vi "io_bin_data_PC_to_instrument.vi"(5 "Binary Data":string, 8 "error in":errorcluster, 10 "Command (none)":string, 11 "VISA resource name":refnum<visa-resource-name>) -> (0 "error out":errorcluster, 3 "VISA resource name out":refnum<visa-resource-name>)   [LabVIEW 2014, in "rszvl_rsidr_core.lvlib"]
uses:
  rszvl_rsidr_core.lvlib
  type_Error_Codes.ctl
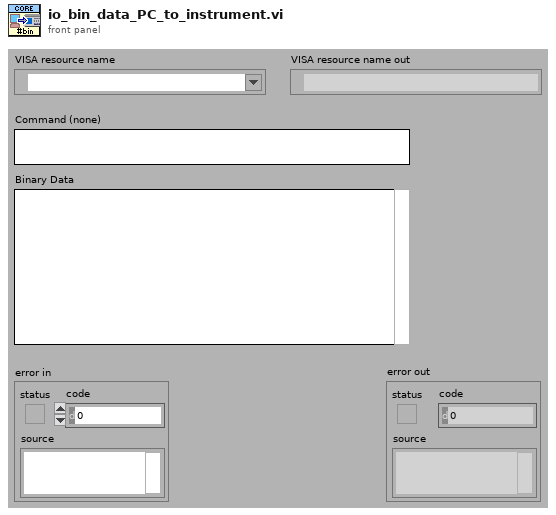
[diagram p1: front panel]
types:
  T1 = typedef "rszvl_rsidr_core.lvlib/type_Error_Codes.ctl" = enum16{"No_error", "VISA_err_ResourceNotFound", "VISA_err_Timeout", "VISA_warn_MoreDataAvailable", "RS_err_MissingCallback", "RS_err_InvalidAttribute", "RS_err_InvalidValue", "RS_err_UnknownResource", "RS_err_AlreadyInitialized", "RS_err_InstrumentStatus", "RS_err_BadRepCapName", "RS_err_TypesMismatch", "RS_err_ValueNotSupported", "RS_err_InvalidRngTable", "RS_err_IDqueryFail", "RS_err_UnexpResponse", "VISA_warn_ConfigNotLoaded", "RS_err_AttributeNotReadable", "RS_err_AttributeNotWritable", "RS_err_InstrumentType", "RS_err_InstrumentOption", "VISA_err_InvalidSize", "RS_err_ReliabilityIndicator", "VISA_warn_UnknownStatus", "VISA_warn_TermCharRead", "VISA_err_IO_error"}
  T2 = typedef "rszvl_rsidr_core.lvlib/type_Session_Data.ctl" = cluster{"Instr type":string, "Instr type for err. msg.":string, "Installed Options":string[], "OPC Timeout":i32, "Query Instrument Status":bool, "Check Range":bool, "Check Options":bool, "Add LF to Write":bool, "Simulate":bool, "Logging":bool, "Logging params":variant, "Interface Type":enum16{"Unknown", "GPIB", "VXI", "GPIB_VXI", "ASRL", "PXI", "TCPIP", "USB", "SOCKET"}, "Fast Sweep":i32, "AdditionalFlags":i32, "WaitBeforeWrite":i32, "WaitBeforeRead":i32, "BinDataChunkSize":i64}
  T3 = enum16{"Unknown", "GPIB", "VXI", "GPIB_VXI", "ASRL", "PXI", "TCPIP", "USB", "SOCKET"}
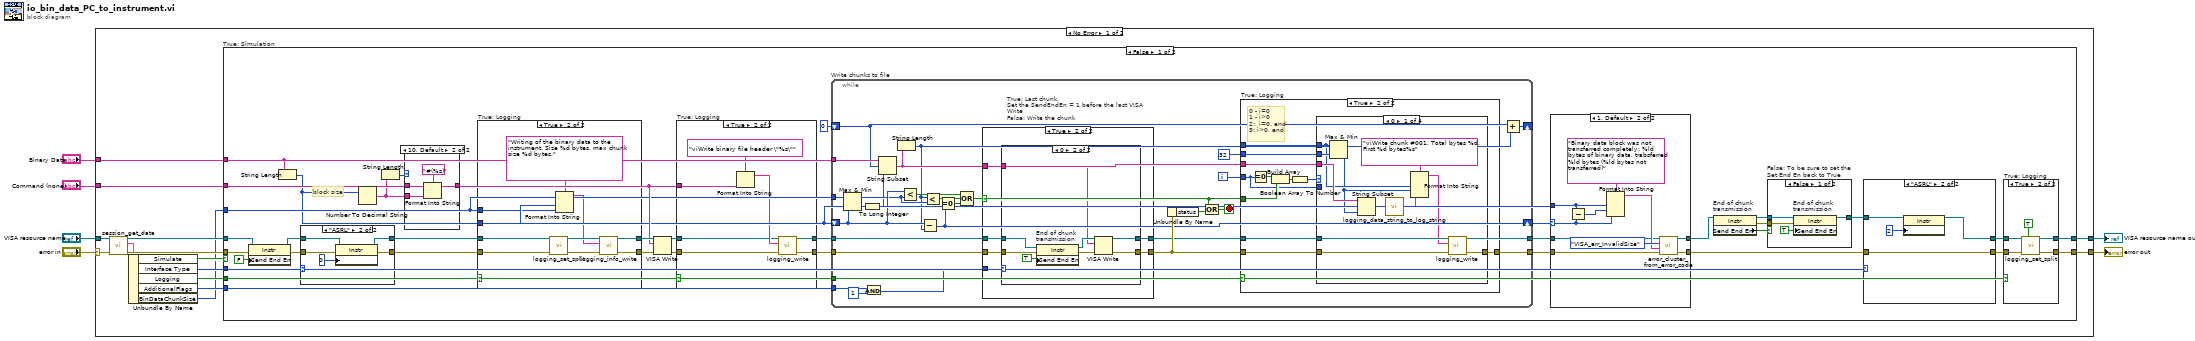
[diagram p0: block diagram]
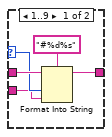
[diagram p7: hidden frame]
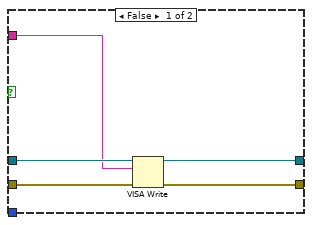
[diagram p8: hidden frame]
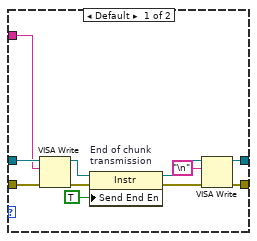
[diagram p9: hidden frame]
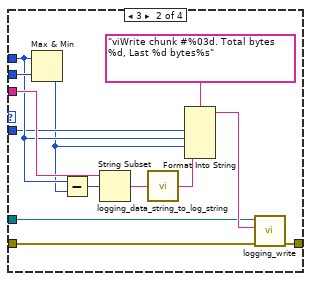
[diagram p11: hidden frame]
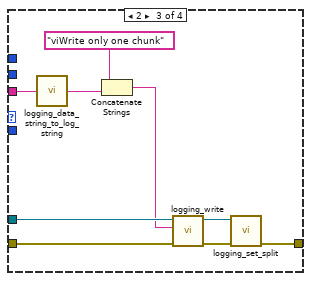
[diagram p12: hidden frame]
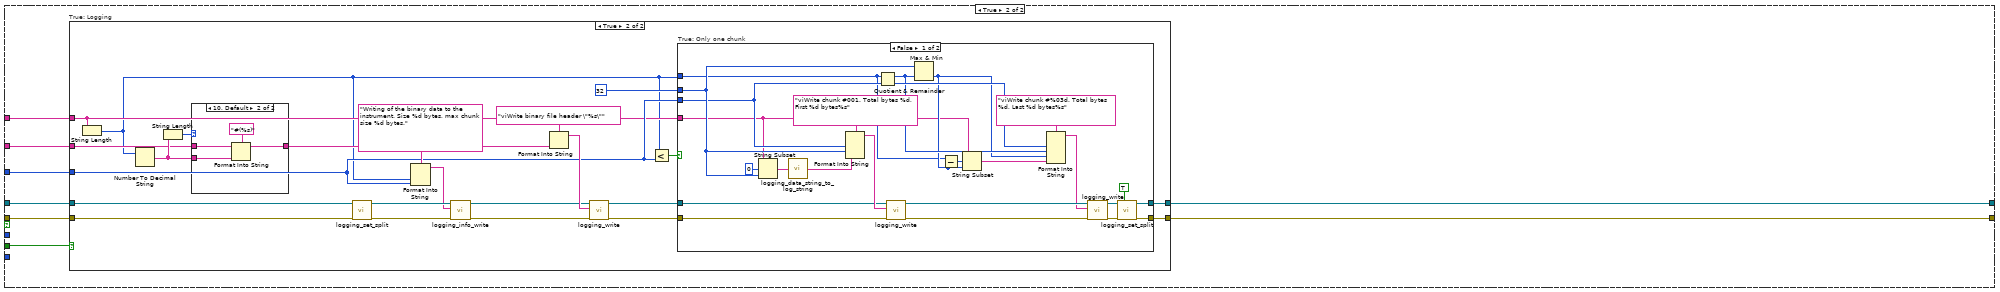
[diagram p16: hidden frame]
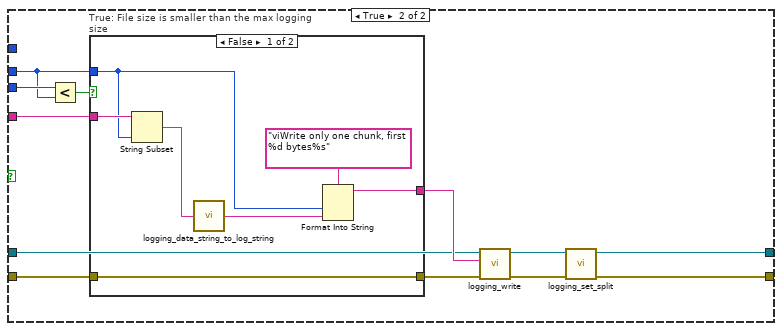
[diagram p18: hidden frame]
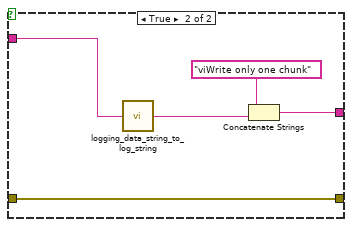
[diagram p19: hidden frame]
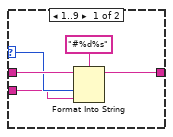
[diagram p20: hidden frame]
diagram:
  n1 = case shown="No Error" "error in" {
    selector: "error in" -> [w18 w319]
    tunnel: "Binary Data" -> [w20 _]
    tunnel: "Command (none)" -> [w19 _]
    tunnel: "VISA resource name" -> [w17 w320]
    tunnel: [w12 w319] -> w3
    tunnel: [w11 w320] -> w2
    frame No Error {
      n2 = call "session_get_data.vi"("error in"=w18, "VISA resource name"=w17) -> ("error out"=w16:errorcluster, "Session User Data out"=w14:T2, "VISA resource name out"=w15:refnum<visa-resource-name>)  [unwired: 7 in]
      n3 = Unbundle By Name(w14) -> ("Simulate"=w10:bool, "Interface Type"=w9:T3, "Logging"=w13:bool, "AdditionalFlags"=w8:i32, "BinDataChunkSize"=w7:i64)
      n4 = case "True: Simulation" shown="False" w10 {
        tunnel: w16 -> [w30 w232]
        tunnel: w15 -> [w57 w231]
        tunnel: w20 -> [w29 w230]
        tunnel: w19 -> [w53 w229]
        tunnel: [w37 w233] -> w11
        tunnel: [w27 w234] -> w12
        tunnel: w13 -> [w40 w235]
        tunnel: w7 -> [w41 w228]
        tunnel: w9 -> [w32 _]
        tunnel: w8 -> [w31 _]
        frame False {
          # "block size"
          n5 = property on="Property Node" class="Instr"(reference=w57, error in=w30, "Send End En"=FALSE ("Message Based Settings:Send End Enable")) -> (reference out=w54:refnum<visa-resource-name>, error out=w55:errorcluster)
          n6 = String Length(string=w29) -> (length=w21:i32)
          n7 = case "4: ASRL" shown="\"ASRL\"" w32 {
            tunnel: w55 -> [w221 w226]
            tunnel: w54 -> [w222 w225]
            tunnel: [w222 w224] -> w50
            tunnel: [w221 w223] -> w49
            frame Default {
            }
            frame "ASRL" {
              n8 = property on="Property Node" class="Instr"(reference=w225, error in=w226, "Serial Settings:End Mode for Reads"=u16 0 ("ASRL End In")) -> (reference out=w224:refnum<visa-resource-name>, error out=w223:errorcluster)
            }
          }
          n9 = Number To Decimal String(number=w21) -> (decimal integer string=w52:string)  [unwired: 1 in]
          n10 = String Length(string=w52) -> (length=w51:i32)
          n11 = case shown="10, Default" w51 {
            selector: w51 -> [w105 _]
            tunnel: w53 -> [w106 w110]
            tunnel: w52 -> [w104 w108]
            tunnel: [w103 w109] -> w43
            frame 1..9 {
              n12 = Format Into String(format string="#%d%s", initial string=w106, w105, w104) -> (resulting string=w103:string)  [unwired: 1 in, 1 out]
            }
            frame 10, Default {
              n13 = Format Into String(format string="#(%s)", initial string=w110, w108) -> (resulting string=w109:string)  [unwired: 1 in, 1 out]
            }
          }
          n14 = case "True: Logging" shown="True" w40 {
            tunnel: w49 -> [w92 w102]
            tunnel: w50 -> [w91 w101]
            tunnel: w41 -> [_ w98]
            tunnel: [w92 w95] -> w47
            tunnel: [w91 w94] -> w48
            tunnel: w21 -> [_ w99]
            frame False {
            }
            frame True {
              n15 = call "logging_set_split.vi"("error in"=w102, "VISA resource name"=w101) -> ("error out"=w97:errorcluster, "VISA resource name out"=w96:refnum<visa-resource-name>)  [unwired: 8 in]
              n16 = Format Into String(format string="Writing of the binary data to the instrument. Size %d bytes, max chunk size %d bytes.", w99, w98) -> (resulting string=w93:string)  [unwired: 2 in, 1 out]
              n17 = call "logging_info_write.vi"("error in"=w97, "String to write"=w93, "VISA resource name"=w96) -> ("error out"=w95:errorcluster, "VISA resource name out"=w94:refnum<visa-resource-name>)  [unwired: 7 in]
            }
          }
          n18 = VISA Write(VISA resource name=w48, write buffer=w43, error in (no error)=w47) -> (VISA resource name out=w45:refnum<visa-resource-name>, error out=w46:errorcluster)  [unwired: 1 out]
          n19 = case "True: Logging" shown="True" w40 {
            tunnel: w46 -> [w83 w88]
            tunnel: w45 -> [w82 w87]
            tunnel: [w83 w86] -> w44
            tunnel: [w82 w85] -> w42
            tunnel: w43 -> [_ w84]
            frame False {
            }
            frame True {
              n20 = Format Into String(format string="viWrite binary file header \"%s\"", w84) -> (resulting string=w89:string)  [unwired: 2 in, 1 out]
              n21 = call "logging_write.vi"("error in"=w88, "String to write"=w89, "VISA resource name"=w87) -> ("error out"=w86:errorcluster, "VISA resource name out"=w85:refnum<visa-resource-name>)  [unwired: 7 in]
            }
          }
          n22 = while "Write chunks to file" {
            tunnel: w44 -> [w118]
            tunnel: w42 -> [w127]
            tunnel: w41 -> [w134]
            shift-right: [w113] -> w25
            shift-left: w21 -> [w136]
            tunnel: [w133] -> w24
            tunnel: w40 -> [w131]
            tunnel: [w125] -> w26
            tunnel: w31 -> [w122]
            tunnel: w29 -> [w120]
            shift-right: [w116] -> _
            shift-left: 0 -> [w115]
            i -> [w128]
            stop <- w137 stop-if-true
            n23 = Max & Min(x=w134, y=w136) -> (min(x,y)=w135:i64)  [unwired: 1 out]
            n24 = To Long Integer(number=w135) -> (32bit integer=w119:i32)
            n25 = And(x=w122, y=1 ("x")) -> (x .and. y?=w121:i32)
            n26 = String Subset(string=w120, offset (0)=w115, length (rest)=w119) -> (substring=w117:string)
            n27 = String Length(string=w117) -> (length=w114:i32)
            n28 = Less?(x=w136, y=w134) -> (x < y?=w130:bool)
            n29 = Subtract(x=w136, y=w114) -> (x-y=w113:i32)
            n30 = Less?(x=w114, y=w134) -> (x < y?=w129:bool)
            n31 = Equal To 0?(x=w113) -> (x = 0?=w112:bool)
            n32 = Compound Arithmetic op=OR(w130, w129, w112) -> (w124:bool)
            n33 = case "True: Last chunk,\nSet the SendEndEn = 1 before the last VISA Write\nFalse: Write the chunk" shown="True" w124 {
              tunnel: w127 -> [w142 w149]
              tunnel: w118 -> [w143 w148]
              tunnel: [w141 w147] -> w126
              tunnel: w117 -> [w139 w146]
              tunnel: [w140 w145] -> w125
              tunnel: w121 -> [_ w144]
              frame False {
                n34 = VISA Write(VISA resource name=w142, write buffer=w139, error in (no error)=w143) -> (VISA resource name out=w140:refnum<visa-resource-name>, error out=w141:errorcluster)  [unwired: 1 out]
              }
              frame True {
                n35 = case shown="0" w144 {
                  tunnel: w149 -> [w154 w168]
                  tunnel: w148 -> [w155 w167]
                  tunnel: [w158 w164] -> w147
                  tunnel: w146 -> [w151 w163]
                  tunnel: [w157 w162] -> w145
                  frame Default {
                    n36 = VISA Write(VISA resource name=w154, write buffer=w151, error in (no error)=w155) -> (VISA resource name out=w152:refnum<visa-resource-name>, error out=w153:errorcluster)  [unwired: 1 out]
                    n37 = property on="End of chunk\ntransmission" class="Instr"(reference=w152, error in=w153, "Send End En"=TRUE ("Message Based Settings:Send End Enable")) -> (reference out=w159:refnum<visa-resource-name>, error out=w160:errorcluster)
                    n38 = VISA Write(VISA resource name=w159, write buffer="\n" ("Line Feed Constant"), error in (no error)=w160) -> (VISA resource name out=w157:refnum<visa-resource-name>, error out=w158:errorcluster)  [unwired: 1 out]
                  }
                  frame 0 {
                    n39 = property on="End of chunk\ntransmission" class="Instr"(reference=w168, error in=w167, "Send End En"=TRUE ("Message Based Settings:Send End Enable")) -> (reference out=w165:refnum<visa-resource-name>, error out=w166:errorcluster)
                    n40 = VISA Write(VISA resource name=w165, write buffer=w163, error in (no error)=w166) -> (VISA resource name out=w162:refnum<visa-resource-name>, error out=w164:errorcluster)  [unwired: 1 out]
                  }
                }
              }
            }
            n41 = Unbundle By Name(w126) -> ("status"=w138:bool)
            n42 = Compound Arithmetic op=OR(w124, w138) -> (w137:bool)
            n43 = case "True: Logging" shown="True" w131 {
              tunnel: w126 -> [w169 w180]
              tunnel: w125 -> [_ w179]
              tunnel: [w169 w178] -> w133
              tunnel: w117 -> [_ w177]
              tunnel: w114 -> [_ w176]
              tunnel: 32 ("length (rest)") -> [_ w175]
              tunnel: w124 -> [_ w174]
              tunnel: w128 -> [_ w170]
              frame False {
              }
              frame True {
                # "0 - i=0\n1 - i>0\n2:  i=0, end\n3: i>0, end"
                n44 = Equal To 0?(x=w170) -> (x = 0?=w173:bool)
                n45 = Build Array(w173, w174) -> (w172:bool[])
                n46 = Boolean Array To Number(Boolean array=w172) -> (number=w171:u32)
                n47 = case shown="0" w171 {
                  tunnel: w180 -> [w189 w202 w213 w214]
                  tunnel: w179 -> [w188 w201 w212 _]
                  tunnel: [w187 w192 w205 w214] -> w178
                  tunnel: w177 -> [w186 w200 w211 _]
                  tunnel: w176 -> [w183 w197 _ _]
                  tunnel: w175 -> [w184 w198 _ _]
                  tunnel: w170 -> [_ w195 _ _]
                  frame 0 {
                    n48 = Max & Min(x=w183, y=w184) -> (min(x,y)=w182:i32)  [unwired: 1 out]
                    n49 = String Subset(string=w186, length (rest)=w182) -> (substring=w185:string)  [unwired: 1 in]
                    n50 = call "logging_data_string_to_log_string.vi"("Raw string to log"=w185) -> ("Result log string"=w181:string)  [unwired: 4 in]
                    n51 = Format Into String(format string="viWrite chunk #001. Total bytes %d, First %d bytes%s", w183, w182, w181) -> (resulting string=w190:string)  [unwired: 2 in, 1 out]
                    n52 = call "logging_write.vi"("error in"=w189, "String to write"=w190, "VISA resource name"=w188) -> ("error out"=w187:errorcluster)  [unwired: 7 in, 1 out]
                  }
                  frame 3 {
                    n53 = Max & Min(x=w197, y=w198) -> (min(x,y)=w194:i32)  [unwired: 1 out]
                    n54 = Subtract(x=w197, y=w194) -> (x-y=w196:i32)
                    n55 = String Subset(string=w200, offset (0)=w196) -> (substring=w199:string)  [unwired: 1 in]
                    n56 = call "logging_data_string_to_log_string.vi"("Raw string to log"=w199) -> ("Result log string"=w193:string)  [unwired: 4 in]
                    n57 = Format Into String(format string="viWrite chunk #%03d. Total bytes %d, Last %d bytes%s", w195, w197, w194, w193) -> (resulting string=w203:string)  [unwired: 2 in, 1 out]
                    n58 = call "logging_write.vi"("error in"=w202, "String to write"=w203, "VISA resource name"=w201) -> ("error out"=w192:errorcluster)  [unwired: 7 in, 1 out]
                  }
                  frame 2 {
                    n59 = call "logging_data_string_to_log_string.vi"("Raw string to log"=w211) -> ("Result log string"=w208:string)  [unwired: 4 in]
                    n60 = Concatenate Strings("viWrite only one chunk" ("format string"), w208) -> (w209:string)
                    n61 = call "logging_write.vi"("error in"=w213, "String to write"=w209, "VISA resource name"=w212) -> ("error out"=w207:errorcluster, "VISA resource name out"=w206:refnum<visa-resource-name>)  [unwired: 7 in]
                    n62 = call "logging_set_split.vi"("error in"=w207, "VISA resource name"=w206) -> ("error out"=w205:errorcluster)  [unwired: 8 in, 1 out]
                  }
                  frame Default {
                  }
                }
              }
            }
            n63 = Add(x=w115, y=w114) -> (x+y=w116:i32)
          }
          n64 = case shown="1, Default" w25 {
            selector: w25 -> [_ w61]
            tunnel: w26 -> [w59 w65]
            tunnel: w24 -> [w58 w64]
            tunnel: [w58 w63] -> w23
            tunnel: [w59 w62] -> w22
            tunnel: w21 -> [_ w60]
            frame 0 {
            }
            frame 1, Default {
              n65 = Subtract(x=w60, y=w61) -> (x-y=w67:i32)
              n66 = Format Into String(format string="Binary data block was not transferred completely: %ld bytes of binary data, trabsferred %ld bytes (%ld bytes not transferred)" ("error message (\"\")"), w60, w67, w61) -> (resulting string=w68:string)  [unwired: 2 in, 1 out]
              n67 = call "error_cluster_from_error_code.vi"("error in"=w64, "error message (\"\")"=w68, "Error Enum in"=type_Error_Codes."VISA_err_InvalidSize", "VISA resource name"=w65) -> ("error out"=w63:errorcluster, "VISA resource name out"=w62:refnum<visa-resource-name>)  [unwired: 6 in]
            }
          }
          n68 = property on="End of chunk\ntransmission" class="Instr"(reference=w22) -> (reference out=w36:refnum<visa-resource-name>, error out=w34:errorcluster, "Send End En"=w35:bool)  [unwired: 1 in]
          n69 = case "False: To be sure to set the\nSet End En back to True" shown="False" w35 {
            tunnel: w36 -> [w73 w74]
            tunnel: w34 -> [w72 _]
            tunnel: [w71 w74] -> w33
            frame False {
              n70 = property on="End of chunk\ntransmission" class="Instr"(reference=w73, error in=w72, "Send End En"=TRUE ("Message Based Settings:Send End Enable")) -> (reference out=w71:refnum<visa-resource-name>)  [unwired: 1 out]
            }
            frame True {
            }
          }
          n71 = case "4: ASRL" shown="\"ASRL\"" w32 {
            tunnel: w33 -> [w215 w219]
            tunnel: [w215 w217] -> w38
            tunnel: w23 -> [w216 w218]
            tunnel: [w216 w218] -> w39
            frame Default {
            }
            frame "ASRL" {
              n72 = property on="Property Node" class="Instr"(reference=w219, "Serial Settings:End Mode for Reads"=u16 2 ("ASRL End In")) -> (reference out=w217:refnum<visa-resource-name>)  [unwired: 1 in, 1 out]
            }
          }
          n73 = case "True: Logging" shown="True" w40 {
            tunnel: w39 -> [w76 w81]
            tunnel: w38 -> [w75 w80]
            tunnel: [w76 w79] -> w27
            tunnel: [w75 w78] -> w37
            frame False {
            }
            frame True {
              n74 = call "logging_set_split.vi"("Evaluate section error (F)"=TRUE, "error in"=w81, "VISA resource name"=w80) -> ("error out"=w79:errorcluster, "VISA resource name out"=w78:refnum<visa-resource-name>)  [unwired: 7 in]
            }
          }
        }
        frame True {
          n75 = case "True: Logging" shown="True" w235 {
            tunnel: w232 -> [w237 w240]
            tunnel: w231 -> [w236 w255]
            tunnel: [w237 w242] -> w234
            tunnel: [w236 w241] -> w233
            tunnel: w230 -> [_ w239]
            tunnel: w229 -> [_ w258]
            tunnel: w228 -> [_ w245]
            frame False {
            }
            frame True {
              n76 = String Length(string=w239) -> (length=w238:i32)
              n77 = Number To Decimal String(number=w238) -> (decimal integer string=w260:string)  [unwired: 1 in]
              n78 = String Length(string=w260) -> (length=w259:i32)
              n79 = case shown="10, Default" w259 {
                selector: w259 -> [w312 _]
                tunnel: w258 -> [w313 w317]
                tunnel: w260 -> [w311 w315]
                tunnel: [w310 w316] -> w248
                frame 1..9 {
                  n80 = Format Into String(format string="#%d%s", initial string=w313, w312, w311) -> (resulting string=w310:string)  [unwired: 1 in, 1 out]
                }
                frame 10, Default {
                  n81 = Format Into String(format string="#(%s)", initial string=w317, w315) -> (resulting string=w316:string)  [unwired: 1 in, 1 out]
                }
              }
              n82 = call "logging_set_split.vi"("error in"=w240, "VISA resource name"=w255) -> ("error out"=w256:errorcluster, "VISA resource name out"=w257:refnum<visa-resource-name>)  [unwired: 8 in]
              n83 = Format Into String(format string="Writing of the binary data to the instrument. Size %d bytes, max chunk size %d bytes.", w238, w245) -> (resulting string=w253:string)  [unwired: 2 in, 1 out]
              n84 = call "logging_info_write.vi"("error in"=w256, "String to write"=w253, "VISA resource name"=w257) -> ("error out"=w250:errorcluster, "VISA resource name out"=w249:refnum<visa-resource-name>)  [unwired: 7 in]
              n85 = Format Into String(format string="viWrite binary file header \"%s\"", w248) -> (resulting string=w251:string)  [unwired: 2 in, 1 out]
              n86 = call "logging_write.vi"("error in"=w250, "String to write"=w251, "VISA resource name"=w249) -> ("error out"=w244:errorcluster, "VISA resource name out"=w243:refnum<visa-resource-name>)  [unwired: 7 in]
              n87 = Less?(x=w238, y=w245) -> (x < y?=w247:bool)
              n88 = case "True: Only one chunk" shown="False" w247 {
                tunnel: 32 ("length (rest)") -> [w278 w290]
                tunnel: w239 -> [w263 w297]
                tunnel: w244 -> [w267 w293]
                tunnel: w245 -> [w277 w296]
                tunnel: w243 -> [w281 w291]
                tunnel: [w271 w287] -> w242
                tunnel: [w270 w286] -> w241
                tunnel: w238 -> [w264 _]
                frame False {
                  n89 = String Subset(string=w263, offset (0)=0, length (rest)=w278) -> (substring=w284:string)
                  n90 = call "logging_data_string_to_log_string.vi"("Raw string to log"=w284) -> ("Result log string"=w285:string)  [unwired: 4 in]
                  n91 = Format Into String(format string="viWrite chunk #001. Total bytes %d, First %d bytes%s", w277, w278, w285) -> (resulting string=w283:string)  [unwired: 2 in, 1 out]
                  n92 = Quotient & Remainder(x=w264, y=w277) -> (x-y*floor(x/y)=w274:i64, floor(x/y)=w275:i64)
                  n93 = call "logging_write.vi"("error in"=w267, "String to write"=w283, "VISA resource name"=w281) -> ("error out"=w262:errorcluster, "VISA resource name out"=w280:refnum<visa-resource-name>)  [unwired: 7 in]
                  n94 = Max & Min(x=w278, y=w274) -> (min(x,y)=w265:i64)  [unwired: 1 out]
                  n95 = Subtract(x=w264, y=w265) -> (x-y=w266:i64)
                  n96 = String Subset(string=w263, offset (0)=w266, length (rest)=w265) -> (substring=w261:string)
                  n97 = Format Into String(format string="viWrite chunk #%03d. Total bytes %d, Last %d bytes%s", w275, w274, w265, w261) -> (resulting string=w276:string)  [unwired: 2 in, 1 out]
                  n98 = call "logging_write.vi"("error in"=w262, "String to write"=w276, "VISA resource name"=w280) -> ("error out"=w273:errorcluster, "VISA resource name out"=w272:refnum<visa-resource-name>)  [unwired: 7 in]
                  n99 = call "logging_set_split.vi"("Evaluate section error (F)"=TRUE, "error in"=w273, "VISA resource name"=w272) -> ("error out"=w271:errorcluster, "VISA resource name out"=w270:refnum<visa-resource-name>)  [unwired: 7 in]
                }
                frame True {
                  n100 = Less?(x=w296, y=w290) -> (x < y?=w295:bool)
                  n101 = case "True: File size is smaller than the max logging size" shown="False" w295 {
                    tunnel: w297 -> [w300 w305]
                    tunnel: [w303 w307] -> w294
                    tunnel: w293 -> [w301 w306]
                    tunnel: [w301 w306] -> w292
                    tunnel: w290 -> [w298 _]
                    frame False {
                      n102 = String Subset(string=w300, length (rest)=w298) -> (substring=w299:string)  [unwired: 1 in]
                      n103 = call "logging_data_string_to_log_string.vi"("Raw string to log"=w299) -> ("Result log string"=w302:string)  [unwired: 4 in]
                      n104 = Format Into String(format string="viWrite only one chunk, first %d bytes%s", w298, w302) -> (resulting string=w303:string)  [unwired: 2 in, 1 out]
                    }
                    frame True {
                      n105 = call "logging_data_string_to_log_string.vi"("Raw string to log"=w305) -> ("Result log string"=w308:string)  [unwired: 4 in]
                      n106 = Concatenate Strings("viWrite only one chunk" ("format string"), w308) -> (w307:string)
                    }
                  }
                  n107 = call "logging_write.vi"("error in"=w292, "String to write"=w294, "VISA resource name"=w291) -> ("error out"=w289:errorcluster, "VISA resource name out"=w288:refnum<visa-resource-name>)  [unwired: 7 in]
                  n108 = call "logging_set_split.vi"("error in"=w289, "VISA resource name"=w288) -> ("error out"=w287:errorcluster, "VISA resource name out"=w286:refnum<visa-resource-name>)  [unwired: 8 in]
                }
              }
            }
          }
        }
      }
    }
    frame Error {
    }
  }
  "error out" <- w3
  "VISA resource name out" <- w2
